vi "LV86_MaskImage.vi"(2 "Mask in":T1 {"Dialogs" format="%.0b"}, 3 "Image":T1 {"Dialogs" format="%.0b"}) -> (1 "Image Out":T1 {"Dialogs" format="%.0b"})   [LabVIEW 2024]
doc: "This vi will mask an image. It will mask all planes or each individual color plane of a color image depending on which poly selection is chosen."
uses:
  <userlib>/ImageProcessing/QTLIB_2595_LV86/QT_Image.ctl
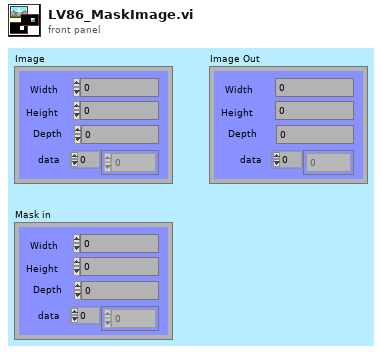
[diagram p1: front panel]
types:
  T1 = typedef "QT_Image.ctl" = cluster{"Width":i32, "Height":i32, "Depth":i32, "data":u8[], "Compressed data":u8[], "Color table":u32[], "Duration":i32, "Options":i32, "Timestamp":i32, "ID":i32, "Reserved":i32, "Dialogs":u32}
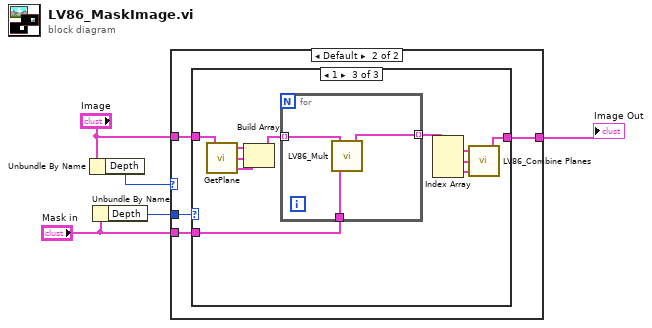
[diagram p0: block diagram]
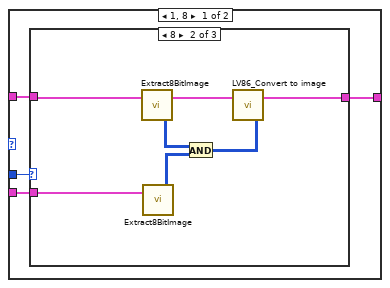
[diagram p2: hidden frame]
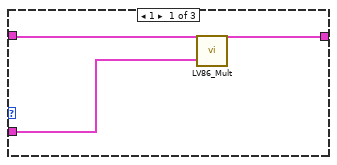
[diagram p3: hidden frame]
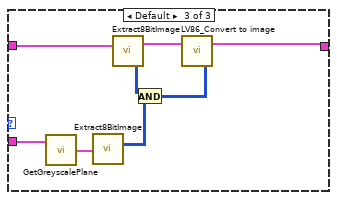
[diagram p4: hidden frame]
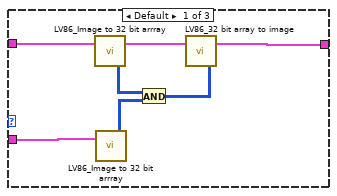
[diagram p5: hidden frame]
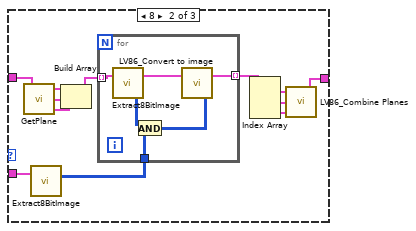
[diagram p6: hidden frame]
diagram:
  n1 = Unbundle By Name("Image") -> ("Depth"=w3:i32)
  n2 = Unbundle By Name("Mask in") -> ("Depth"=w1:i32)
  n3 = case shown="Default" w3 {
    tunnel: "Mask in" -> [w9 w31]
    tunnel: [w8 w30] -> w5
    tunnel: "Image" -> [w7 w29]
    tunnel: w1 -> [w6 w28]
    frame 1, 8 {
      n4 = case shown="8" w6 {
        tunnel: w9 -> [w11 w19 w22]
        tunnel: [w10 w18 w20] -> w8
        tunnel: w7 -> [w12 w13 w23]
        frame 1 {
          n5 = call <userlib>:"LV86_Mult.vi"("Image 2"=w11, "Image"=w12) -> ("Image Out"=w10:T1)  [unwired: 1 in]
        }
        frame 8 {
          n6 = call <userlib>:"Extract8BitImage.vi"("Image in"=w13) -> ("Intensity Graph"=w17:u8[][], "Image out"=w15:T1)  [unwired: 1 in]
          n7 = call <userlib>:"Extract8BitImage.vi"("Image in"=w19) -> ("Intensity Graph"=w16:u8[][])  [unwired: 1 in, 1 out]
          n8 = And(x=w17, y=w16) -> (x .and. y?=w14:u8[][])
          n9 = call <userlib>:"LV86_Convert to image.vi"("Intensity Graph"=w14, "Image In"=w15) -> ("Image Out"=w18:T1)  [unwired: 1 in]
        }
        frame Default {
          n10 = call <userlib>:"GetGreyscalePlane.vi"("Image In"=w22) -> ("Greyscale  Out"=w21:T1)
          n11 = call <userlib>:"Extract8BitImage.vi"("Image in"=w21) -> ("Intensity Graph"=w27:u8[][])  [unwired: 1 in, 1 out]
          n12 = call <userlib>:"Extract8BitImage.vi"("Image in"=w23) -> ("Intensity Graph"=w26:u8[][], "Image out"=w25:T1)  [unwired: 1 in]
          n13 = And(x=w26, y=w27) -> (x .and. y?=w24:u8[][])
          n14 = call <userlib>:"LV86_Convert to image.vi"("Intensity Graph"=w24, "Image In"=w25) -> ("Image Out"=w20:T1)  [unwired: 1 in]
        }
      }
    }
    frame Default {
      n15 = case shown="1" w28 {
        tunnel: w31 -> [w38 w50 w57]
        tunnel: [w37 w39 w58] -> w30
        tunnel: w29 -> [w32 w48 w67]
        frame Default {
          n16 = call <userlib>:"LV86_Image to 32 bit arrray.vi"("Image In"=w32) -> ("Intensity Graph"=w36:u32[][], "Image out"=w34:T1)  [unwired: 1 in]
          n17 = call <userlib>:"LV86_Image to 32 bit arrray.vi"("Image In"=w38) -> ("Intensity Graph"=w35:u32[][])  [unwired: 1 in, 1 out]
          n18 = And(x=w36, y=w35) -> (x .and. y?=w33:u32[][])
          n19 = call <userlib>:"LV86_32 bit array to image.vi"("Intensity Graph"=w33, "Image In"=w34) -> ("Image Out"=w37:T1)  [unwired: 1 in]
        }
        frame 8 {
          n20 = call <userlib>:"GetPlane.vi"("Image In"=w48) -> ("Blue Plane Out"=w44:T1, "Green Plane Out"=w45:T1, "Red Plane Out"=w46:T1)
          n21 = call <userlib>:"Extract8BitImage.vi"("Image in"=w50) -> ("Intensity Graph"=w49:u8[][])  [unwired: 1 in, 1 out]
          n22 = Build Array(w46, w45, w44) -> (w47:T1[])
          n23 = for {
            tunnel: [w56] -> w43 mode=indexing
            tunnel: w49 -> [w54]
            tunnel: w47 -> [w51] mode=indexing
            n24 = call <userlib>:"Extract8BitImage.vi"("Image in"=w51) -> ("Intensity Graph"=w55:u8[][], "Image out"=w53:T1)  [unwired: 1 in]
            n25 = And(x=w55, y=w54) -> (x .and. y?=w52:u8[][])
            n26 = call <userlib>:"LV86_Convert to image.vi"("Intensity Graph"=w52, "Image In"=w53) -> ("Image Out"=w56:T1)  [unwired: 1 in]
          }
          n27 = Index Array(array=w43) -> (element #1=w42:T1, element #2=w41:T1, element #3=w40:T1)  [unwired: 3 in]
          n28 = call <userlib>:"LV86_Combine Planes.vi"("Blue"=w40, "Green"=w41, "Red"=w42) -> ("Image 2"=w39:T1)  [unwired: 1 in]
        }
        frame 1 {
          n29 = call <userlib>:"GetPlane.vi"("Image In"=w67) -> ("Blue Plane Out"=w63:T1, "Green Plane Out"=w64:T1, "Red Plane Out"=w65:T1)
          n30 = Build Array(w65, w64, w63) -> (w66:T1[])
          n31 = for {
            tunnel: [w68] -> w62 mode=indexing
            tunnel: w66 -> [w70] mode=indexing
            tunnel: w57 -> [w69]
            n32 = call <userlib>:"LV86_Mult.vi"("Image 2"=w69, "Image"=w70) -> ("Image Out"=w68:T1)  [unwired: 1 in]
          }
          n33 = Index Array(array=w62) -> (element #1=w61:T1, element #2=w60:T1, element #3=w59:T1)  [unwired: 3 in]
          n34 = call <userlib>:"LV86_Combine Planes.vi"("Blue"=w59, "Green"=w60, "Red"=w61) -> ("Image 2"=w58:T1)  [unwired: 1 in]
        }
      }
    }
  }
  "Image Out" <- w5
